vi "configurePerChannel.vi"(8 "error in (no error)":errorcluster, 10 "physical channels":string, 11 "A66xxSupply in":refnum<class "A66xxSupply.lvclass">) -> (0 "error out":errorcluster, 3 "A66xxSupply out":refnum<class "A66xxSupply.lvclass">)   [LabVIEW 2011, in "Hardware.lvlib" / "Channels.lvlib" / "A66xxSupply.lvclass"]
uses:
  A66xxSupply.lvclass
  AnalogOutput.lvclass
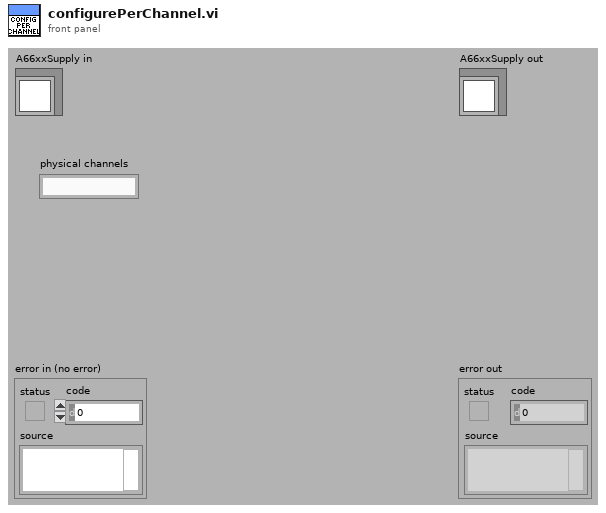
[diagram p1: front panel]
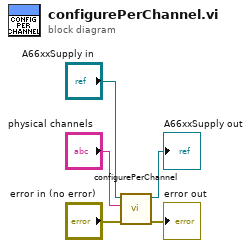
[diagram p0: block diagram]
diagram:
  n1 = call-parent "configurePerChannel.vi"("error in (no error)"="error in (no error)", "physical channels"="physical channels", "AnalogOutput in"="A66xxSupply in") -> ("error out"=→"error out":errorcluster, "AnalogOutput out"=→"A66xxSupply out":refnum<class "A66xxSupply.lvclass">)  [unwired: 7 in]
